vi "QPlus_Lockin_Analyzer_beta.vi"() -> ()   [LabVIEW 2016]
uses:
  <instrlib>/Stanford Research 830/Public/Data/Read (1 Parameter).vi
  <vilib>/Utility/file.llb/Write Delimited Spreadsheet (DBL).vi
  <instrlib>/Stanford Research 830/Stanford Research 830.lvlib
panel:
  out "FWHM":dbl
  out "Quality Factor":dbl
  out "Integrated Signal":cluster{"Y":dbl[], "Y":dbl[]}[](graph)
  out "Resonance Frequency":dbl
  in  "VISA resource name":refnum<visa-resource-name>
  in  "Sensitivity (26: 1 V/uA)":i8(ring)=26 items=["Auto Gain"=-1, "2 nV/fA"=0, "5 nV/fA"=1, "10 nV/fA"=2, "20 nV/fA"=3, "50 nV/fA"=4, "100 nV/fA"=5, "200 nV/fA"=6, "500 nV/fA"=7, "1 uV/pA"=8, "2 uV/pA"=9, "5 uV/pA"=10, "10 uV/pA"=11, "20 uV/pA"=12, "50 uV/pA"=13, "100 uV/pA"=14, "200 uV/pA"=15, "500 uV/pA"=16, "1 mV/nA"=17, "2 mV/nA"=18, "5 mV/nA"=19, "10 mV/nA"=20, "20 mV/nA"=21, "50 mV/nA"=22, "100 mV/nA"=23, "200 mV/nA"=24, "500 mV/mA"=25, "1 V/uA"=26]
  in  "Time Constant (8: 100ms)":u16(ring)=8 items=["10 us", "30 us", "100 us", "300 us", "1 ms", "3 ms", "10 ms", "30 ms", "100 ms", "300 ms", "1 s", "3 s", "10 s", "30 s", "100 s", "300 s", "1 ks", "3 ks", "10 ks", "30 ks"]
  out "Raw Signal":cluster{"Y":dbl[], "Y":dbl[]}[](graph)
  in  "Save File Name":path=path "G:/UCB/Instruments/tip making/Qplus AFM tip making/qplus test/Caihong/CJ39.xlsx" caption="Filename"
  in  "Time Between Points (sec)":dbl=0.05 format="%#_1f"
  in  "Sine Output Amplitude (1 V)":dbl=1.0
  in  "Starting Frequency (Hz)":dbl=32000.0
  in  "Final Frequency (Hz)":dbl=33000.0
  in  "Step Size (Hz)":dbl=10.0
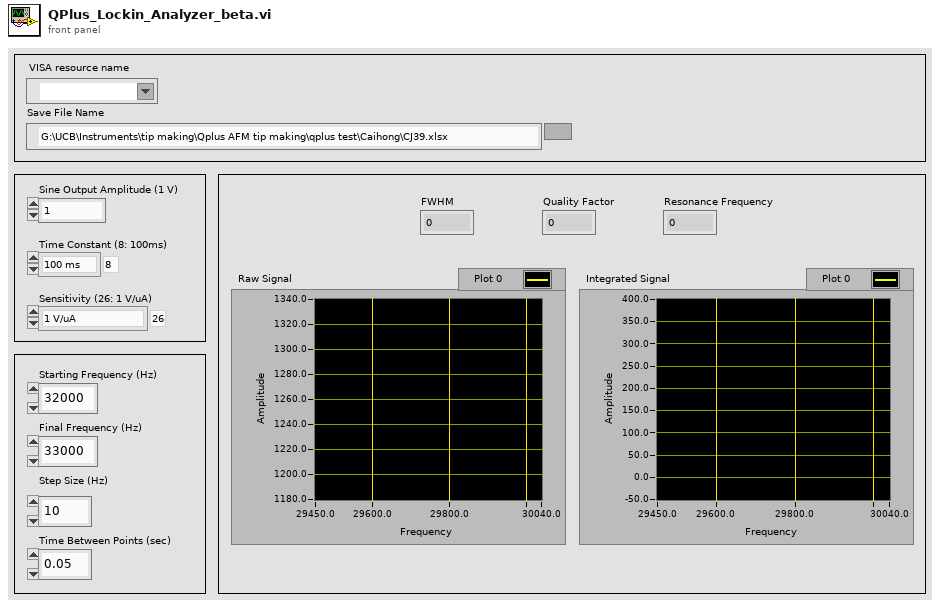
[diagram p1: front panel]
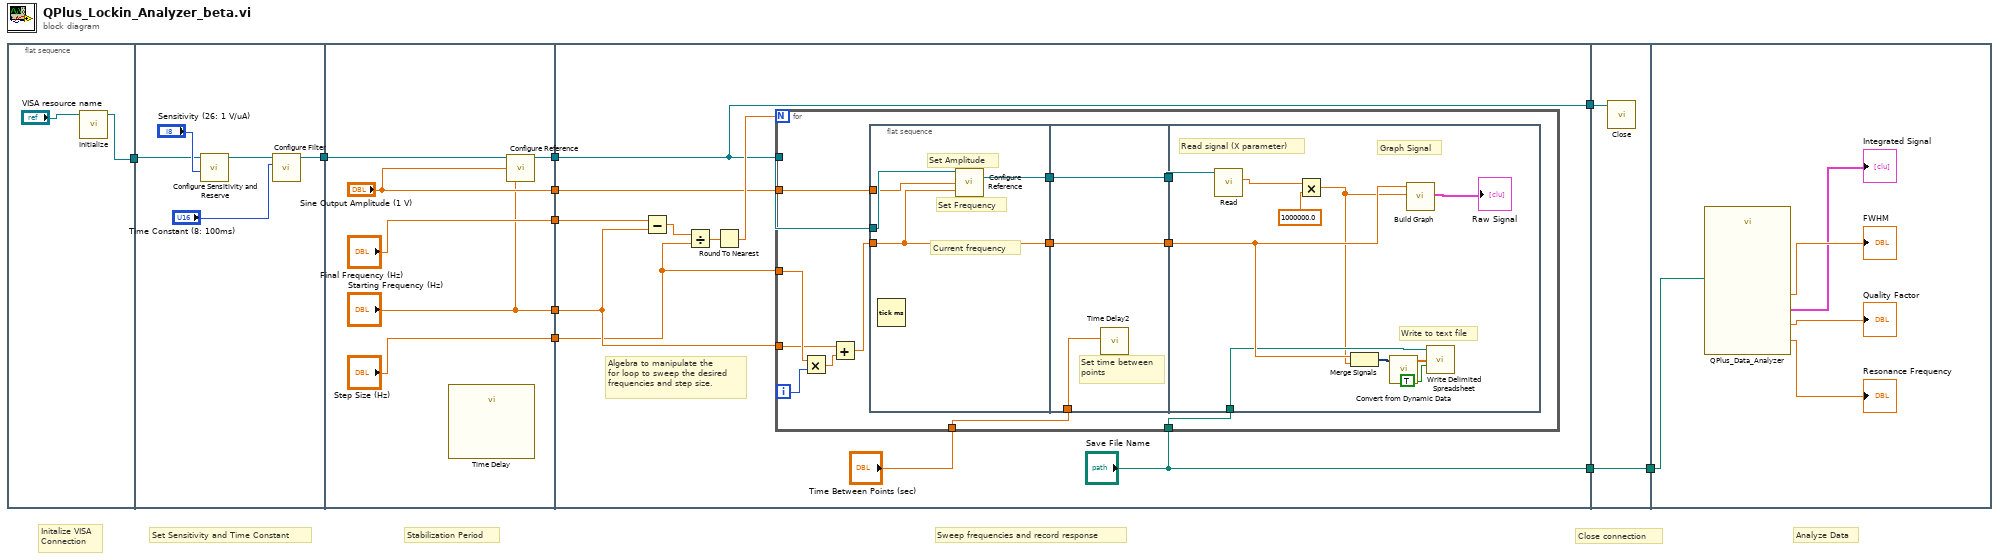
[diagram p0: block diagram]
diagram:
  # "Stabilization Period"
  # "Analyze Data"
  # "Close connection"
  # "Sweep frequencies and record response"
  # "Set Sensitivity and Time Constant"
  # "Initalize VISA\nConnection"
  n1 = flat-sequence {
    tunnel: [w11] -> w10
    tunnel: [w14] -> w6
    tunnel: w10 -> [w13]
    tunnel: w6 -> [w23]
    tunnel: [w22] -> w5
    tunnel: ["Starting Frequency (Hz)"] -> w4
    tunnel: ["Final Frequency (Hz)"] -> w3
    tunnel: ["Step Size (Hz)"] -> w2
    tunnel: ["Sine Output Amplitude (1 V)"] -> w1
    tunnel: w5 -> [w30]
    tunnel: [w30] -> w9
    tunnel: ["Save File Name"] -> w8
    tunnel: w4 -> [w27]
    tunnel: w3 -> [w26]
    tunnel: w2 -> [w25]
    tunnel: w1 -> [w24]
    tunnel: w9 -> [w65]
    tunnel: w8 -> [w64]
    tunnel: [w64] -> w7
    tunnel: w7 -> [w70]
    frame #0 {
      n2 = call <instrlib>:"Initialize.vi"("VISA resource name"="VISA resource name") -> ("VISA resource name out"=w11:refnum<visa-resource-name>)  [unwired: 9 in, 1 out]
    }
    frame #1 {
      n3 = call <instrlib>:"Configure Sensitivity and Reserve.vi"("Sensitivity (-1: Auto gain)"="Sensitivity (26: 1 V/uA)", "VISA resource name"=w13) -> ("VISA resource name out"=w16:refnum<visa-resource-name>)  [unwired: 8 in, 1 out]
      n4 = call <instrlib>:"Configure Filter.vi"("Time Constant (8: 100ms)"="Time Constant (8: 100ms)", "VISA resource name"=w16) -> ("VISA resource name out"=w14:refnum<visa-resource-name>)  [unwired: 8 in, 1 out]
    }
    frame #2 {
      n5 = call "Time Delay"() -> ()  [unwired: 11 in, 1 out]
      n6 = call <instrlib>:"Configure Reference.vi"("VISA resource name"=w23, "Sine Output Amplitude (1 V)"="Sine Output Amplitude (1 V)", "Internal Reference Frequency (1000 Hz)"="Starting Frequency (Hz)") -> ("VISA resource name out"=w22:refnum<visa-resource-name>)  [unwired: 11 in, 1 out]
    }
    frame #3 {
      # "Algebra to manipulate the\nfor loop to sweep the desired\nfrequencies and step size."
      n7 = Subtract(x=w26, y=w27) -> (x-y=w33:dbl)
      n8 = Divide(x=w33, y=w25) -> (x/y=w32:dbl)
      n9 = Round To Nearest(number=w32) -> (nearest integer value=w31:dbl)
      n10 = for {
        N: w31 -> [_]
        tunnel: w25 -> [w45]
        tunnel: w27 -> [w43]
        tunnel: w30 -> [w41]
        tunnel: "Time Between Points (sec)" -> [w34]
        tunnel: "Save File Name" -> [w40]
        tunnel: w24 -> [w39]
        i -> [w46]
        n11 = Multiply(x=w45, y=w46) -> (x*y=w44:dbl)
        n12 = Add(x=w43, y=w44) -> (x+y=w42:dbl)
        n13 = flat-sequence {
          tunnel: [w50] -> w38
          tunnel: [w48] -> w36
          tunnel: w42 -> [w48]
          tunnel: w41 -> [w49]
          tunnel: w39 -> [w47]
          tunnel: w38 -> [w53]
          tunnel: [w53] -> w37
          tunnel: w36 -> [w52]
          tunnel: [w52] -> w35
          tunnel: w34 -> [w51]
          tunnel: w37 -> [w59]
          tunnel: w35 -> [w58]
          tunnel: w40 -> [w57]
          frame #0 {
            # "Set Frequency"
            # "Set Amplitude"
            # "Current frequency"
            n14 = Tick Count (ms)() -> ()  [unwired: 1 out]
            n15 = call <instrlib>:"Configure Reference.vi"("VISA resource name"=w49, "Sine Output Amplitude (1 V)"=w47, "Internal Reference Frequency (1000 Hz)"=w48) -> ("VISA resource name out"=w50:refnum<visa-resource-name>)  [unwired: 11 in, 1 out]
          }
          frame #1 {
            # "Set time between\npoints"
            n16 = call "Time Delay2"("Delay Time (s)"=w51) -> ()  [unwired: 10 in, 1 out]
          }
          frame #2 {
            # "Read signal (X parameter)"
            # "Graph Signal"
            # "Write to text file"
            n17 = call-poly <instrlib>:"Read.vi"("VISA resource name"=w59) -> ("Measurement"=w56:dbl)  [unwired: 8 in, 2 out]
            n18 = Multiply(x=w56, y=1000000.0) -> (x*y=w54:dbl)
            n19 = Merge Signals(w58, w54) -> (w61:dynamicdata)
            n20 = call "Convert from Dynamic Data"("Dynamic Data Type"=w61) -> ("Array"=w60:dbl[])  [unwired: 3 in]
            n21 = call "Build Graph"("Y Input"=w54, "X Input"=w58) -> ("XY Graph"=→"Raw Signal":cluster{"Y":dbl[], "Y":dbl[]}[])  [unwired: 3 in, 6 out]
            n22 = call-poly <vilib>:"Write Delimited Spreadsheet.vi"("file path (dialog if empty)"=w57, "1D data"=w60, "append to file? (new file:F)"=TRUE) -> ()  [unwired: 11 in, 2 out]
          }
        }
      }
    }
    frame #4 {
      n23 = call <instrlib>:"Close.vi"("VISA resource name"=w65) -> ()  [unwired: 10 in, 1 out]
    }
    frame #5 {
      n24 = call "QPlus_Data_Analyzer.vi"("File Path"=w70) -> ("Resonance Frequency"=→"Resonance Frequency":dbl, "Quality Factor"=→"Quality Factor":dbl, "FWHM"=→"FWHM":dbl, "Integrated Signal"=→"Integrated Signal":cluster{"Y":dbl[], "Y":dbl[]}[])  [unwired: 7 in]
    }
  }
